vi "loading.vi"(10 "string2":string="勤眾興業", 11 "string1":string="CHEN") -> ()   [LabVIEW 2015]
uses:
  USER32.DLL
panel:
  in  "Color Box 2":u32(colorbox)=56466
  in  "CHEN 2":bool
  out "Cluster 11":T1
  in  "CHEN":bool
  in  "Color Box":u32(colorbox)=46079
  out "Cluster 10":T2
  out "Cluster 9":T3
  out "Cluster 8":T4
  out "Cluster 7":T3
  out "Cluster 6":T3
  out "Cluster 3":T3
  out "Cluster 4":T5
  out "Cluster 2":T6
  out "Cluster":T7
  out "Round Color Box 48":u32(colorbox)
  out "Round Color Box 47":u32(colorbox)
  out "Round Color Box 46":u32(colorbox)
  out "Round Color Box 45":u32(colorbox)
  out "Round Color Box 44":u32(colorbox)
  out "Round Color Box 43":u32(colorbox)
  out "Round Color Box 42":u32(colorbox)
  out "Round Color Box 41":u32(colorbox)
  out "Round Color Box 40":u32(colorbox)
  out "Round Color Box 39":u32(colorbox)
  out "Round Color Box 38":u32(colorbox)
  out "Round Color Box 37":u32(colorbox)
  out "Round Color Box 36":u32(colorbox)
  out "Round Color Box 35":u32(colorbox)
  out "Round Color Box 34":u32(colorbox)
  out "Round Color Box 33":u32(colorbox)
  out "Round Color Box 32":u32(colorbox)
  out "Round Color Box 31":u32(colorbox)
  out "Round Color Box 30":u32(colorbox)
  out "Round Color Box 29":u32(colorbox)
  out "Round Color Box 28":u32(colorbox)
  out "Round Color Box 27":u32(colorbox)
  out "Round Color Box 26":u32(colorbox)
  out "Round Color Box 25":u32(colorbox)
  out "Round Color Box 24":u32(colorbox)
  out "Round Color Box 23":u32(colorbox)
  out "Round Color Box 22":u32(colorbox)
  out "Round Color Box 21":u32(colorbox)
  out "Round Color Box 20":u32(colorbox)
  out "Round Color Box 19":u32(colorbox)
  out "Round Color Box 18":u32(colorbox)
  out "Round Color Box 17":u32(colorbox)
  in  "stop":bool
  out "Round Color Box 16":u32(colorbox)
  out "Round Color Box 15":u32(colorbox)
  out "Round Color Box 14":u32(colorbox)
  out "Round Color Box 13":u32(colorbox)
  out "Round Color Box 12":u32(colorbox)
  out "Round Color Box 11":u32(colorbox)
  out "Round Color Box 10":u32(colorbox)
  out "Round Color Box 9":u32(colorbox)
  out "Round Color Box 8":u32(colorbox)
  out "Round Color Box 7":u32(colorbox)
  out "Round Color Box 6":u32(colorbox)
  out "Round Color Box 5":u32(colorbox)
  out "Round Color Box 4":u32(colorbox)
  out "Round Color Box 3":u32(colorbox)
  out "Round Color Box 2":u32(colorbox)
  out "Round Color Box":u32(colorbox)
  # "Loading..."
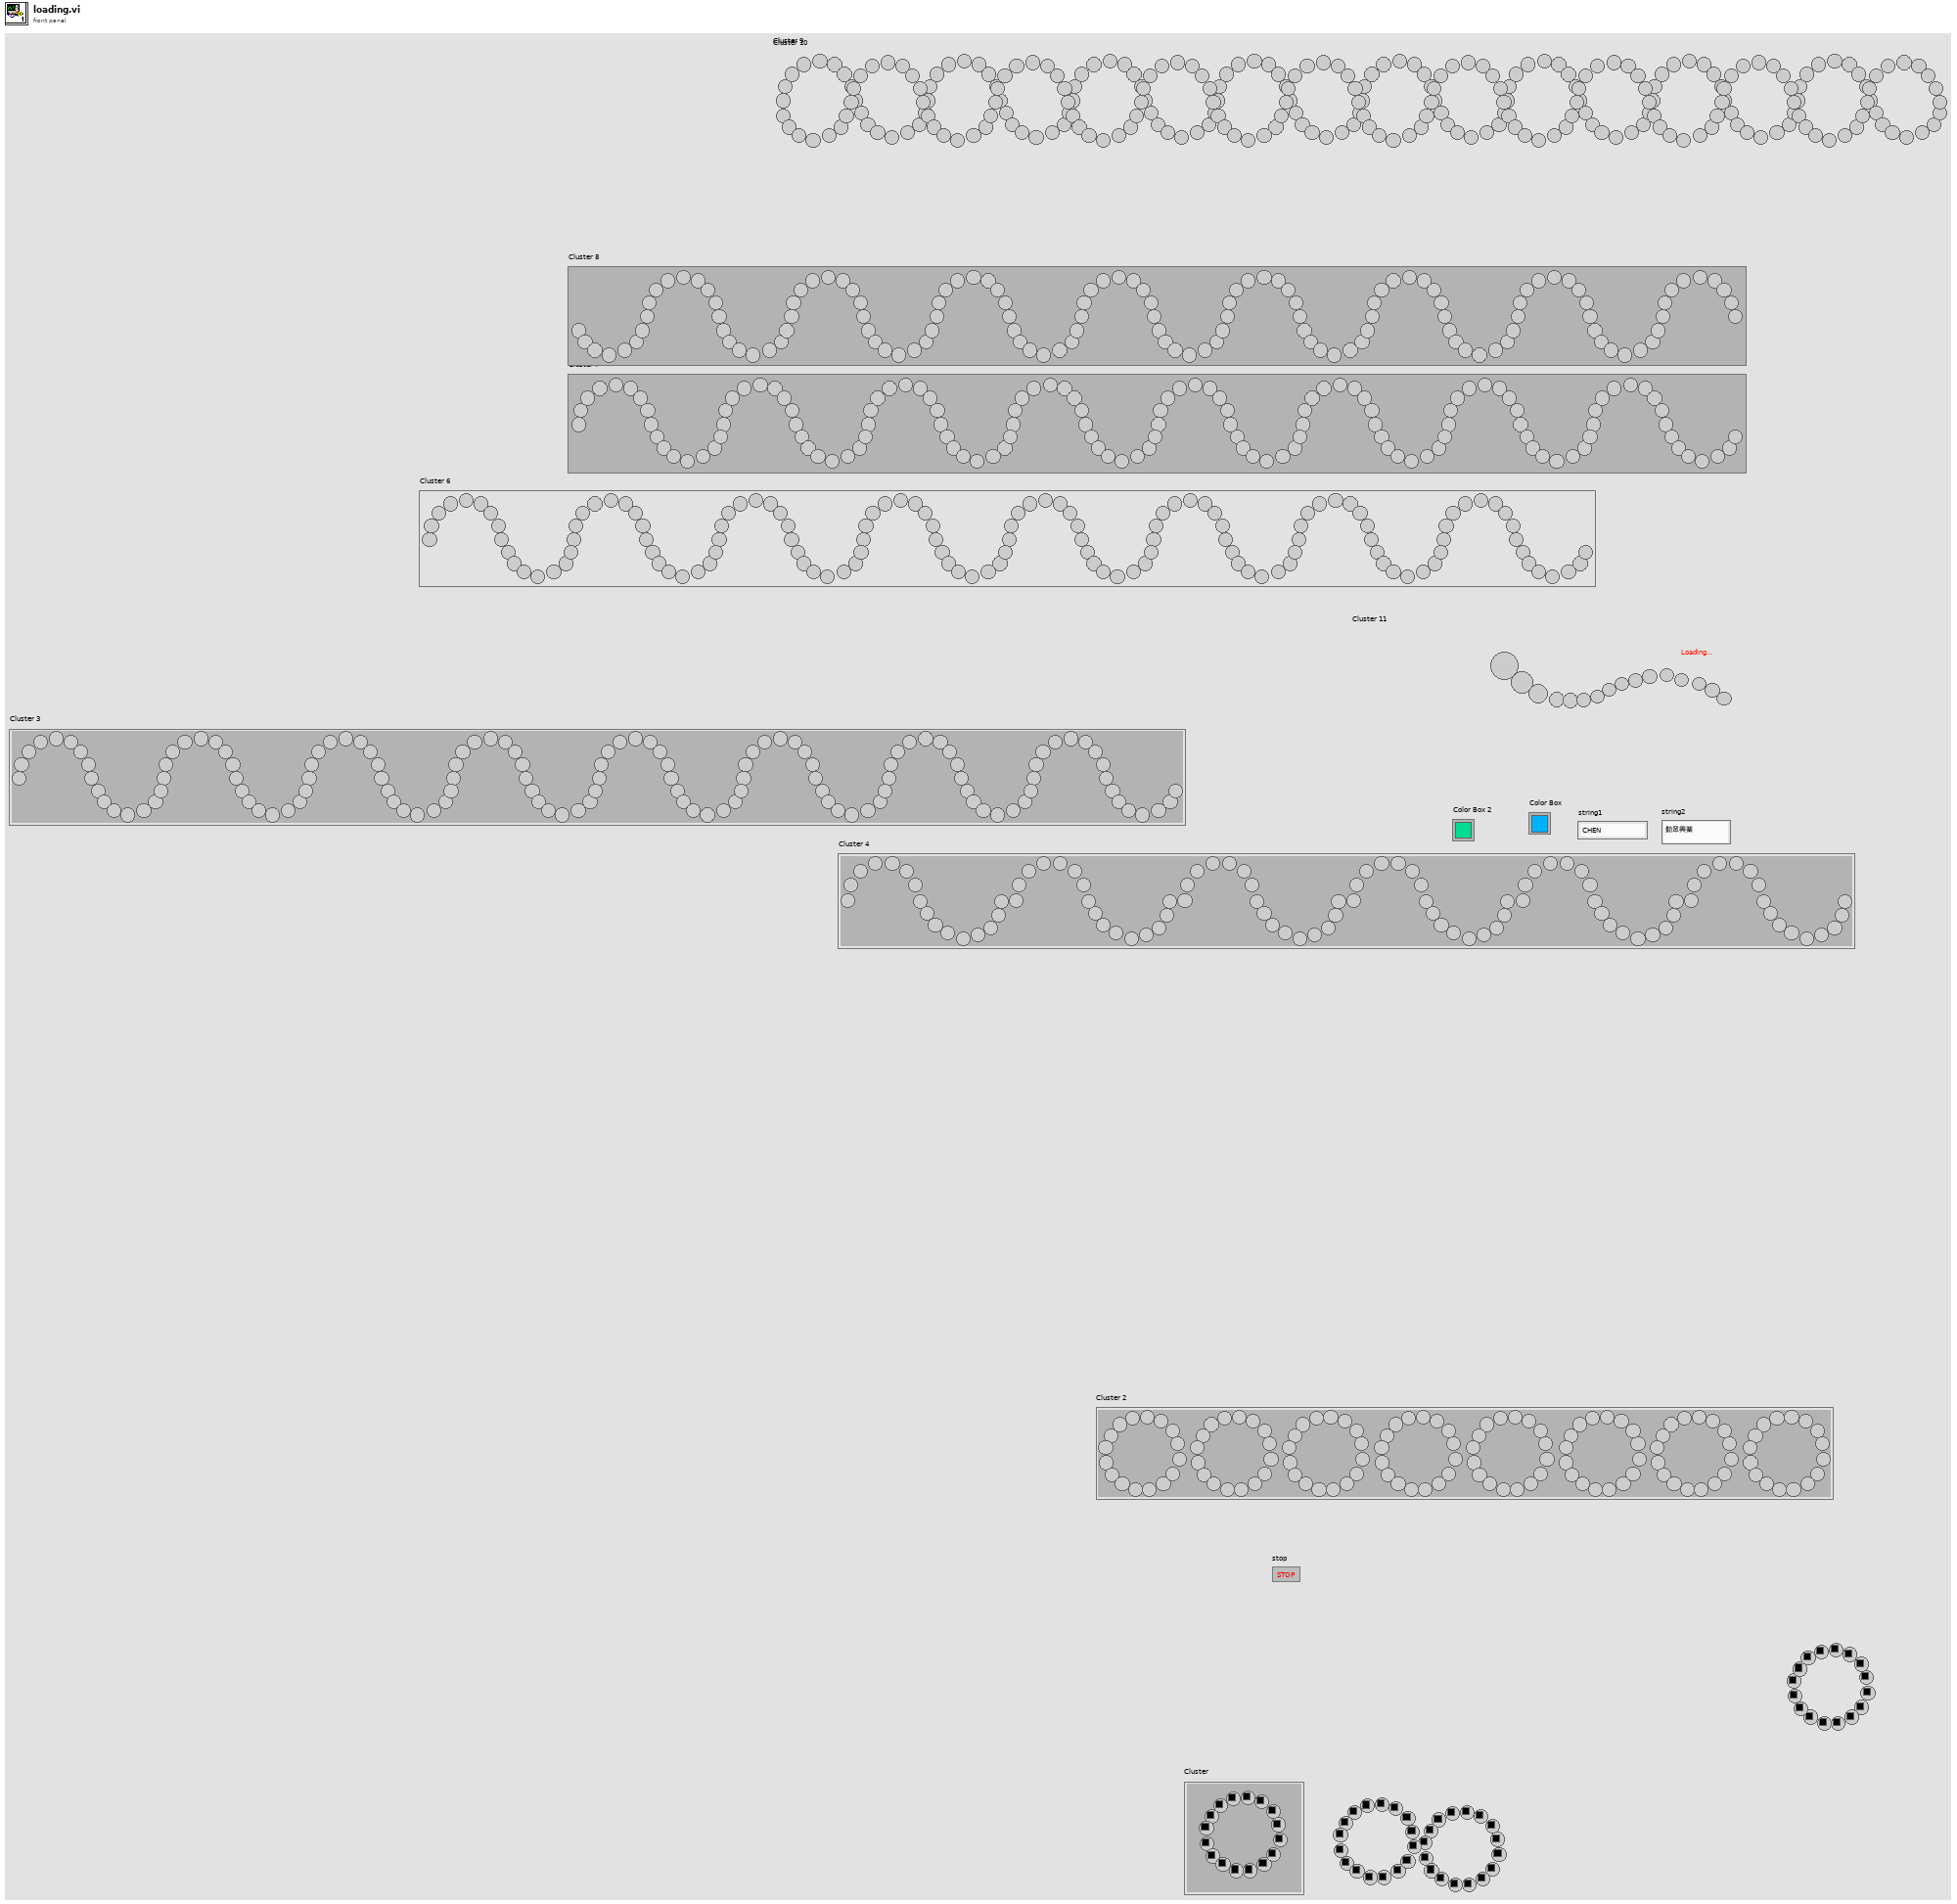
[diagram p1: front panel]
types:
  T1 = cluster{"Round Color Box 72":u32, "Round Color Box 73":u32, "Round Color Box 74":u32, "Round Color Box 75":u32, "Round Color Box 76":u32, "Round Color Box 77":u32, "Round Color Box 78":u32, "Round Color Box 79":u32, "Round Color Box 80":u32, "Round Color Box 65":u32, "Round Color Box 66":u32, "Round Color Box 67":u32, "Round Color Box 68":u32, "Round Color Box 69":u32, "Round Color Box 70":u32, "Round Color Box 71":u32}
  T2 = cluster{"Round Color Box 72":u32, "Round Color Box 73":u32, "Round Color Box 74":u32, "Round Color Box 75":u32, "Round Color Box 76":u32, "Round Color Box 77":u32, "Round Color Box 78":u32, "Round Color Box 79":u32, "Round Color Box 80":u32, "Round Color Box 65":u32, "Round Color Box 66":u32, "Round Color Box 67":u32, "Round Color Box 68":u32, "Round Color Box 69":u32, "Round Color Box 70":u32, "Round Color Box 71":u32, "Round Color Box 88":u32, "Round Color Box 89":u32, "Round Color Box 90":u32, "Round Color Box 91":u32, "Round Color Box 92":u32, "Round Color Box 93":u32, "Round Color Box 94":u32, "Round Color Box 95":u32, "Round Color Box 96":u32, "Round Color Box 81":u32, "Round Color Box 82":u32, "Round Color Box 83":u32, "Round Color Box 84":u32, "Round Color Box 85":u32, "Round Color Box 86":u32, "Round Color Box 87":u32, "Round Color Box 104":u32, "Round Color Box 105":u32, "Round Color Box 106":u32, "Round Color Box 107":u32, "Round Color Box 108":u32, "Round Color Box 109":u32, "Round Color Box 110":u32, "Round Color Box 111":u32, "Round Color Box 112":u32, "Round Color Box 97":u32, "Round Color Box 98":u32, "Round Color Box 99":u32, "Round Color Box 100":u32, "Round Color Box 101":u32, "Round Color Box 102":u32, "Round Color Box 103":u32, "Round Color Box 120":u32, "Round Color Box 121":u32, "Round Color Box 122":u32, "Round Color Box 123":u32, "Round Color Box 124":u32, "Round Color Box 125":u32, "Round Color Box 126":u32, "Round Color Box 127":u32, "Round Color Box 128":u32, "Round Color Box 113":u32, "Round Color Box 114":u32, "Round Color Box 115":u32, "Round Color Box 116":u32, "Round Color Box 117":u32, "Round Color Box 118":u32, "Round Color Box 119":u32, "Round Color Box 136":u32, "Round Color Box 137":u32, "Round Color Box 138":u32, "Round Color Box 139":u32, "Round Color Box 140":u32, "Round Color Box 141":u32, "Round Color Box 142":u32, "Round Color Box 143":u32, "Round Color Box 144":u32, "Round Color Box 129":u32, "Round Color Box 130":u32, "Round Color Box 131":u32, "Round Color Box 132":u32, "Round Color Box 133":u32, "Round Color Box 134":u32, "Round Color Box 135":u32, "Round Color Box 152":u32, "Round Color Box 153":u32, "Round Color Box 154":u32, "Round Color Box 155":u32, "Round Color Box 156":u32, "Round Color Box 157":u32, "Round Color Box 158":u32, "Round Color Box 159":u32, "Round Color Box 160":u32, "Round Color Box 145":u32, "Round Color Box 146":u32, "Round Color Box 147":u32, "Round Color Box 148":u32, "Round Color Box 149":u32, "Round Color Box 150":u32, "Round Color Box 151":u32, "Round Color Box 168":u32, "Round Color Box 169":u32, "Round Color Box 170":u32, "Round Color Box 171":u32, "Round Color Box 172":u32, "Round Color Box 173":u32, "Round Color Box 174":u32, "Round Color Box 175":u32, "Round Color Box 176":u32, "Round Color Box 161":u32, "Round Color Box 162":u32, "Round Color Box 163":u32, "Round Color Box 164":u32, "Round Color Box 165":u32, "Round Color Box 166":u32, "Round Color Box 167":u32, "Round Color Box 184":u32, "Round Color Box 185":u32, "Round Color Box 186":u32, "Round Color Box 187":u32, "Round Color Box 188":u32, "Round Color Box 189":u32, "Round Color Box 190":u32, "Round Color Box 191":u32, "Round Color Box 192":u32, "Round Color Box 177":u32, "Round Color Box 178":u32, "Round Color Box 179":u32, "Round Color Box 180":u32, "Round Color Box 181":u32, "Round Color Box 182":u32, "Round Color Box 183":u32}
  T3 = cluster{"Round Color Box 60":u32, "Round Color Box 59":u32, "Round Color Box 58":u32, "Round Color Box 57":u32, "Round Color Box 56":u32, "Round Color Box 55":u32, "Round Color Box 54":u32, "Round Color Box 53":u32, "Round Color Box 52":u32, "Round Color Box 51":u32, "Round Color Box 50":u32, "Round Color Box 49":u32, "Round Color Box 64":u32, "Round Color Box 63":u32, "Round Color Box 62":u32, "Round Color Box 61":u32, "Round Color Box 65":u32, "Round Color Box 66":u32, "Round Color Box 67":u32, "Round Color Box 68":u32, "Round Color Box 69":u32, "Round Color Box 70":u32, "Round Color Box 71":u32, "Round Color Box 72":u32, "Round Color Box 73":u32, "Round Color Box 74":u32, "Round Color Box 75":u32, "Round Color Box 76":u32, "Round Color Box 77":u32, "Round Color Box 78":u32, "Round Color Box 79":u32, "Round Color Box 80":u32, "Round Color Box 81":u32, "Round Color Box 82":u32, "Round Color Box 83":u32, "Round Color Box 84":u32, "Round Color Box 85":u32, "Round Color Box 86":u32, "Round Color Box 87":u32, "Round Color Box 88":u32, "Round Color Box 89":u32, "Round Color Box 90":u32, "Round Color Box 91":u32, "Round Color Box 92":u32, "Round Color Box 93":u32, "Round Color Box 94":u32, "Round Color Box 95":u32, "Round Color Box 96":u32, "Round Color Box 97":u32, "Round Color Box 98":u32, "Round Color Box 99":u32, "Round Color Box 100":u32, "Round Color Box 101":u32, "Round Color Box 102":u32, "Round Color Box 103":u32, "Round Color Box 104":u32, "Round Color Box 105":u32, "Round Color Box 106":u32, "Round Color Box 107":u32, "Round Color Box 108":u32, "Round Color Box 109":u32, "Round Color Box 110":u32, "Round Color Box 111":u32, "Round Color Box 112":u32, "Round Color Box 113":u32, "Round Color Box 114":u32, "Round Color Box 115":u32, "Round Color Box 116":u32, "Round Color Box 117":u32, "Round Color Box 118":u32, "Round Color Box 119":u32, "Round Color Box 120":u32, "Round Color Box 121":u32, "Round Color Box 122":u32, "Round Color Box 123":u32, "Round Color Box 124":u32, "Round Color Box 125":u32, "Round Color Box 126":u32, "Round Color Box 127":u32, "Round Color Box 128":u32, "Round Color Box 129":u32, "Round Color Box 130":u32, "Round Color Box 131":u32, "Round Color Box 132":u32, "Round Color Box 133":u32, "Round Color Box 134":u32, "Round Color Box 135":u32, "Round Color Box 136":u32, "Round Color Box 137":u32, "Round Color Box 138":u32, "Round Color Box 139":u32, "Round Color Box 140":u32, "Round Color Box 141":u32, "Round Color Box 142":u32, "Round Color Box 143":u32, "Round Color Box 144":u32, "Round Color Box 145":u32, "Round Color Box 146":u32, "Round Color Box 147":u32, "Round Color Box 148":u32, "Round Color Box 149":u32, "Round Color Box 150":u32, "Round Color Box 151":u32, "Round Color Box 152":u32, "Round Color Box 153":u32, "Round Color Box 154":u32, "Round Color Box 155":u32, "Round Color Box 156":u32, "Round Color Box 157":u32, "Round Color Box 158":u32, "Round Color Box 159":u32, "Round Color Box 160":u32, "Round Color Box 161":u32, "Round Color Box 162":u32, "Round Color Box 163":u32, "Round Color Box 164":u32, "Round Color Box 165":u32, "Round Color Box 166":u32, "Round Color Box 167":u32, "Round Color Box 168":u32, "Round Color Box 169":u32, "Round Color Box 170":u32, "Round Color Box 171":u32, "Round Color Box 172":u32, "Round Color Box 173":u32, "Round Color Box 174":u32, "Round Color Box 175":u32, "Round Color Box 176":u32}
  T4 = cluster{"Round Color Box 72":u32, "Round Color Box 73":u32, "Round Color Box 74":u32, "Round Color Box 75":u32, "Round Color Box 76":u32, "Round Color Box 77":u32, "Round Color Box 78":u32, "Round Color Box 79":u32, "Round Color Box 80":u32, "Round Color Box 65":u32, "Round Color Box 66":u32, "Round Color Box 67":u32, "Round Color Box 68":u32, "Round Color Box 69":u32, "Round Color Box 70":u32, "Round Color Box 71":u32, "Round Color Box 81":u32, "Round Color Box 82":u32, "Round Color Box 83":u32, "Round Color Box 84":u32, "Round Color Box 85":u32, "Round Color Box 86":u32, "Round Color Box 87":u32, "Round Color Box 88":u32, "Round Color Box 89":u32, "Round Color Box 90":u32, "Round Color Box 91":u32, "Round Color Box 92":u32, "Round Color Box 93":u32, "Round Color Box 94":u32, "Round Color Box 95":u32, "Round Color Box 96":u32, "Round Color Box 97":u32, "Round Color Box 98":u32, "Round Color Box 99":u32, "Round Color Box 100":u32, "Round Color Box 101":u32, "Round Color Box 102":u32, "Round Color Box 103":u32, "Round Color Box 104":u32, "Round Color Box 105":u32, "Round Color Box 106":u32, "Round Color Box 107":u32, "Round Color Box 108":u32, "Round Color Box 109":u32, "Round Color Box 110":u32, "Round Color Box 111":u32, "Round Color Box 112":u32, "Round Color Box 113":u32, "Round Color Box 114":u32, "Round Color Box 115":u32, "Round Color Box 116":u32, "Round Color Box 117":u32, "Round Color Box 118":u32, "Round Color Box 119":u32, "Round Color Box 120":u32, "Round Color Box 121":u32, "Round Color Box 122":u32, "Round Color Box 123":u32, "Round Color Box 124":u32, "Round Color Box 125":u32, "Round Color Box 126":u32, "Round Color Box 127":u32, "Round Color Box 128":u32, "Round Color Box 129":u32, "Round Color Box 130":u32, "Round Color Box 131":u32, "Round Color Box 132":u32, "Round Color Box 133":u32, "Round Color Box 134":u32, "Round Color Box 135":u32, "Round Color Box 136":u32, "Round Color Box 137":u32, "Round Color Box 138":u32, "Round Color Box 139":u32, "Round Color Box 140":u32, "Round Color Box 141":u32, "Round Color Box 142":u32, "Round Color Box 143":u32, "Round Color Box 144":u32, "Round Color Box 145":u32, "Round Color Box 146":u32, "Round Color Box 147":u32, "Round Color Box 148":u32, "Round Color Box 149":u32, "Round Color Box 150":u32, "Round Color Box 151":u32, "Round Color Box 152":u32, "Round Color Box 153":u32, "Round Color Box 154":u32, "Round Color Box 155":u32, "Round Color Box 156":u32, "Round Color Box 157":u32, "Round Color Box 158":u32, "Round Color Box 159":u32, "Round Color Box 160":u32, "Round Color Box 161":u32, "Round Color Box 162":u32, "Round Color Box 163":u32, "Round Color Box 164":u32, "Round Color Box 165":u32, "Round Color Box 166":u32, "Round Color Box 167":u32, "Round Color Box 168":u32, "Round Color Box 169":u32, "Round Color Box 170":u32, "Round Color Box 171":u32, "Round Color Box 172":u32, "Round Color Box 173":u32, "Round Color Box 174":u32, "Round Color Box 175":u32, "Round Color Box 176":u32, "Round Color Box 177":u32, "Round Color Box 178":u32, "Round Color Box 179":u32, "Round Color Box 180":u32, "Round Color Box 181":u32, "Round Color Box 182":u32, "Round Color Box 183":u32, "Round Color Box 184":u32, "Round Color Box 185":u32, "Round Color Box 186":u32, "Round Color Box 187":u32, "Round Color Box 188":u32, "Round Color Box 189":u32, "Round Color Box 190":u32, "Round Color Box 191":u32, "Round Color Box 192":u32}
  T5 = cluster{"Round Color Box 65":u32, "Round Color Box 66":u32, "Round Color Box 67":u32, "Round Color Box 68":u32, "Round Color Box 69":u32, "Round Color Box 70":u32, "Round Color Box 71":u32, "Round Color Box 72":u32, "Round Color Box 73":u32, "Round Color Box 74":u32, "Round Color Box 75":u32, "Round Color Box 76":u32, "Round Color Box 77":u32, "Round Color Box 78":u32, "Round Color Box 79":u32, "Round Color Box 80":u32, "Round Color Box 81":u32, "Round Color Box 82":u32, "Round Color Box 83":u32, "Round Color Box 84":u32, "Round Color Box 85":u32, "Round Color Box 86":u32, "Round Color Box 87":u32, "Round Color Box 88":u32, "Round Color Box 89":u32, "Round Color Box 90":u32, "Round Color Box 91":u32, "Round Color Box 92":u32, "Round Color Box 93":u32, "Round Color Box 94":u32, "Round Color Box 95":u32, "Round Color Box 96":u32, "Round Color Box 97":u32, "Round Color Box 98":u32, "Round Color Box 99":u32, "Round Color Box 100":u32, "Round Color Box 101":u32, "Round Color Box 102":u32, "Round Color Box 103":u32, "Round Color Box 104":u32, "Round Color Box 105":u32, "Round Color Box 106":u32, "Round Color Box 107":u32, "Round Color Box 108":u32, "Round Color Box 109":u32, "Round Color Box 110":u32, "Round Color Box 111":u32, "Round Color Box 112":u32, "Round Color Box 113":u32, "Round Color Box 114":u32, "Round Color Box 115":u32, "Round Color Box 116":u32, "Round Color Box 117":u32, "Round Color Box 118":u32, "Round Color Box 119":u32, "Round Color Box 120":u32, "Round Color Box 121":u32, "Round Color Box 122":u32, "Round Color Box 123":u32, "Round Color Box 124":u32, "Round Color Box 125":u32, "Round Color Box 126":u32, "Round Color Box 127":u32, "Round Color Box 128":u32, "Round Color Box 129":u32, "Round Color Box 130":u32, "Round Color Box 131":u32, "Round Color Box 132":u32, "Round Color Box 133":u32, "Round Color Box 134":u32, "Round Color Box 135":u32, "Round Color Box 136":u32, "Round Color Box 137":u32, "Round Color Box 138":u32, "Round Color Box 139":u32, "Round Color Box 140":u32, "Round Color Box 141":u32, "Round Color Box 142":u32, "Round Color Box 143":u32, "Round Color Box 144":u32, "Round Color Box 145":u32, "Round Color Box 146":u32, "Round Color Box 147":u32, "Round Color Box 148":u32, "Round Color Box 149":u32, "Round Color Box 150":u32, "Round Color Box 151":u32, "Round Color Box 152":u32, "Round Color Box 153":u32, "Round Color Box 154":u32, "Round Color Box 155":u32, "Round Color Box 156":u32, "Round Color Box 157":u32, "Round Color Box 158":u32, "Round Color Box 159":u32, "Round Color Box 160":u32}
  T6 = cluster{"Round Color Box 49":u32, "Round Color Box 50":u32, "Round Color Box 51":u32, "Round Color Box 52":u32, "Round Color Box 53":u32, "Round Color Box 54":u32, "Round Color Box 55":u32, "Round Color Box 56":u32, "Round Color Box 57":u32, "Round Color Box 58":u32, "Round Color Box 59":u32, "Round Color Box 60":u32, "Round Color Box 61":u32, "Round Color Box 62":u32, "Round Color Box 63":u32, "Round Color Box 64":u32, "Round Color Box 65":u32, "Round Color Box 66":u32, "Round Color Box 67":u32, "Round Color Box 68":u32, "Round Color Box 69":u32, "Round Color Box 70":u32, "Round Color Box 71":u32, "Round Color Box 72":u32, "Round Color Box 73":u32, "Round Color Box 74":u32, "Round Color Box 75":u32, "Round Color Box 76":u32, "Round Color Box 77":u32, "Round Color Box 78":u32, "Round Color Box 79":u32, "Round Color Box 80":u32, "Round Color Box 81":u32, "Round Color Box 82":u32, "Round Color Box 83":u32, "Round Color Box 84":u32, "Round Color Box 85":u32, "Round Color Box 86":u32, "Round Color Box 87":u32, "Round Color Box 88":u32, "Round Color Box 89":u32, "Round Color Box 90":u32, "Round Color Box 91":u32, "Round Color Box 92":u32, "Round Color Box 93":u32, "Round Color Box 94":u32, "Round Color Box 95":u32, "Round Color Box 96":u32, "Round Color Box 97":u32, "Round Color Box 98":u32, "Round Color Box 99":u32, "Round Color Box 100":u32, "Round Color Box 101":u32, "Round Color Box 102":u32, "Round Color Box 103":u32, "Round Color Box 104":u32, "Round Color Box 105":u32, "Round Color Box 106":u32, "Round Color Box 107":u32, "Round Color Box 108":u32, "Round Color Box 109":u32, "Round Color Box 110":u32, "Round Color Box 111":u32, "Round Color Box 112":u32, "Round Color Box 113":u32, "Round Color Box 114":u32, "Round Color Box 115":u32, "Round Color Box 116":u32, "Round Color Box 117":u32, "Round Color Box 118":u32, "Round Color Box 119":u32, "Round Color Box 120":u32, "Round Color Box 121":u32, "Round Color Box 122":u32, "Round Color Box 123":u32, "Round Color Box 124":u32, "Round Color Box 125":u32, "Round Color Box 126":u32, "Round Color Box 127":u32, "Round Color Box 128":u32, "Round Color Box 129":u32, "Round Color Box 130":u32, "Round Color Box 131":u32, "Round Color Box 132":u32, "Round Color Box 133":u32, "Round Color Box 134":u32, "Round Color Box 135":u32, "Round Color Box 136":u32, "Round Color Box 137":u32, "Round Color Box 138":u32, "Round Color Box 139":u32, "Round Color Box 140":u32, "Round Color Box 141":u32, "Round Color Box 142":u32, "Round Color Box 143":u32, "Round Color Box 144":u32, "Round Color Box 145":u32, "Round Color Box 146":u32, "Round Color Box 147":u32, "Round Color Box 148":u32, "Round Color Box 149":u32, "Round Color Box 150":u32, "Round Color Box 151":u32, "Round Color Box 152":u32, "Round Color Box 153":u32, "Round Color Box 154":u32, "Round Color Box 155":u32, "Round Color Box 156":u32, "Round Color Box 157":u32, "Round Color Box 158":u32, "Round Color Box 159":u32, "Round Color Box 160":u32, "Round Color Box 161":u32, "Round Color Box 162":u32, "Round Color Box 163":u32, "Round Color Box 164":u32, "Round Color Box 165":u32, "Round Color Box 166":u32, "Round Color Box 167":u32, "Round Color Box 168":u32, "Round Color Box 169":u32, "Round Color Box 170":u32, "Round Color Box 171":u32, "Round Color Box 172":u32, "Round Color Box 173":u32, "Round Color Box 174":u32, "Round Color Box 175":u32, "Round Color Box 176":u32}
  T7 = cluster{"Round Color Box 49":u32, "Round Color Box 50":u32, "Round Color Box 51":u32, "Round Color Box 52":u32, "Round Color Box 53":u32, "Round Color Box 54":u32, "Round Color Box 55":u32, "Round Color Box 56":u32, "Round Color Box 57":u32, "Round Color Box 58":u32, "Round Color Box 59":u32, "Round Color Box 60":u32, "Round Color Box 61":u32, "Round Color Box 62":u32, "Round Color Box 63":u32, "Round Color Box 64":u32}
  T8 = cluster{"Round Color Box":u32, "Round Color Box 2":u32, "Round Color Box 3":u32, "Round Color Box 4":u32, "Round Color Box 5":u32, "Round Color Box 6":u32, "Round Color Box 7":u32, "Round Color Box 8":u32, "Round Color Box 9":u32, "Round Color Box 10":u32, "Round Color Box 11":u32, "Round Color Box 12":u32, "Round Color Box 13":u32, "Round Color Box 14":u32, "Round Color Box 15":u32, "Round Color Box 16":u32}
  T9 = cluster{"[0]":u32, "[1]":u32, "[2]":u32, "[3]":u32, "[4]":u32, "[5]":u32, "[6]":u32, "[7]":u32, "[8]":u32, "[9]":u32, "[10]":u32, "[11]":u32, "[12]":u32, "[13]":u32, "[14]":u32, "[15]":u32}
  T10 = enum8{"Enabled", "Disabled", "Disabled and Grayed Out"}
  T11 = cluster{"[0]":u32, "[1]":u32, "[2]":u32, "[3]":u32, "[4]":u32, "[5]":u32, "[6]":u32, "[7]":u32, "[8]":u32, "[9]":u32, "[10]":u32, "[11]":u32, "[12]":u32, "[13]":u32, "[14]":u32, "[15]":u32, "[16]":u32, "[17]":u32, "[18]":u32, "[19]":u32, "[20]":u32, "[21]":u32, "[22]":u32, "[23]":u32, "[24]":u32, "[25]":u32, "[26]":u32, "[27]":u32, "[28]":u32, "[29]":u32, "[30]":u32, "[31]":u32, "[32]":u32, "[33]":u32, "[34]":u32, "[35]":u32, "[36]":u32, "[37]":u32, "[38]":u32, "[39]":u32, "[40]":u32, "[41]":u32, "[42]":u32, "[43]":u32, "[44]":u32, "[45]":u32, "[46]":u32, "[47]":u32, "[48]":u32, "[49]":u32, "[50]":u32, "[51]":u32, "[52]":u32, "[53]":u32, "[54]":u32, "[55]":u32, "[56]":u32, "[57]":u32, "[58]":u32, "[59]":u32, "[60]":u32, "[61]":u32, "[62]":u32, "[63]":u32, "[64]":u32, "[65]":u32, "[66]":u32, "[67]":u32, "[68]":u32, "[69]":u32, "[70]":u32, "[71]":u32, "[72]":u32, "[73]":u32, "[74]":u32, "[75]":u32, "[76]":u32, "[77]":u32, "[78]":u32, "[79]":u32, "[80]":u32, "[81]":u32, "[82]":u32, "[83]":u32, "[84]":u32, "[85]":u32, "[86]":u32, "[87]":u32, "[88]":u32, "[89]":u32, "[90]":u32, "[91]":u32, "[92]":u32, "[93]":u32, "[94]":u32, "[95]":u32, "[96]":u32, "[97]":u32, "[98]":u32, "[99]":u32, "[100]":u32, "[101]":u32, "[102]":u32, "[103]":u32, "[104]":u32, "[105]":u32, "[106]":u32, "[107]":u32, "[108]":u32, "[109]":u32, "[110]":u32, "[111]":u32, "[112]":u32, "[113]":u32, "[114]":u32, "[115]":u32, "[116]":u32, "[117]":u32, "[118]":u32, "[119]":u32, "[120]":u32, "[121]":u32, "[122]":u32, "[123]":u32, "[124]":u32, "[125]":u32, "[126]":u32, "[127]":u32}
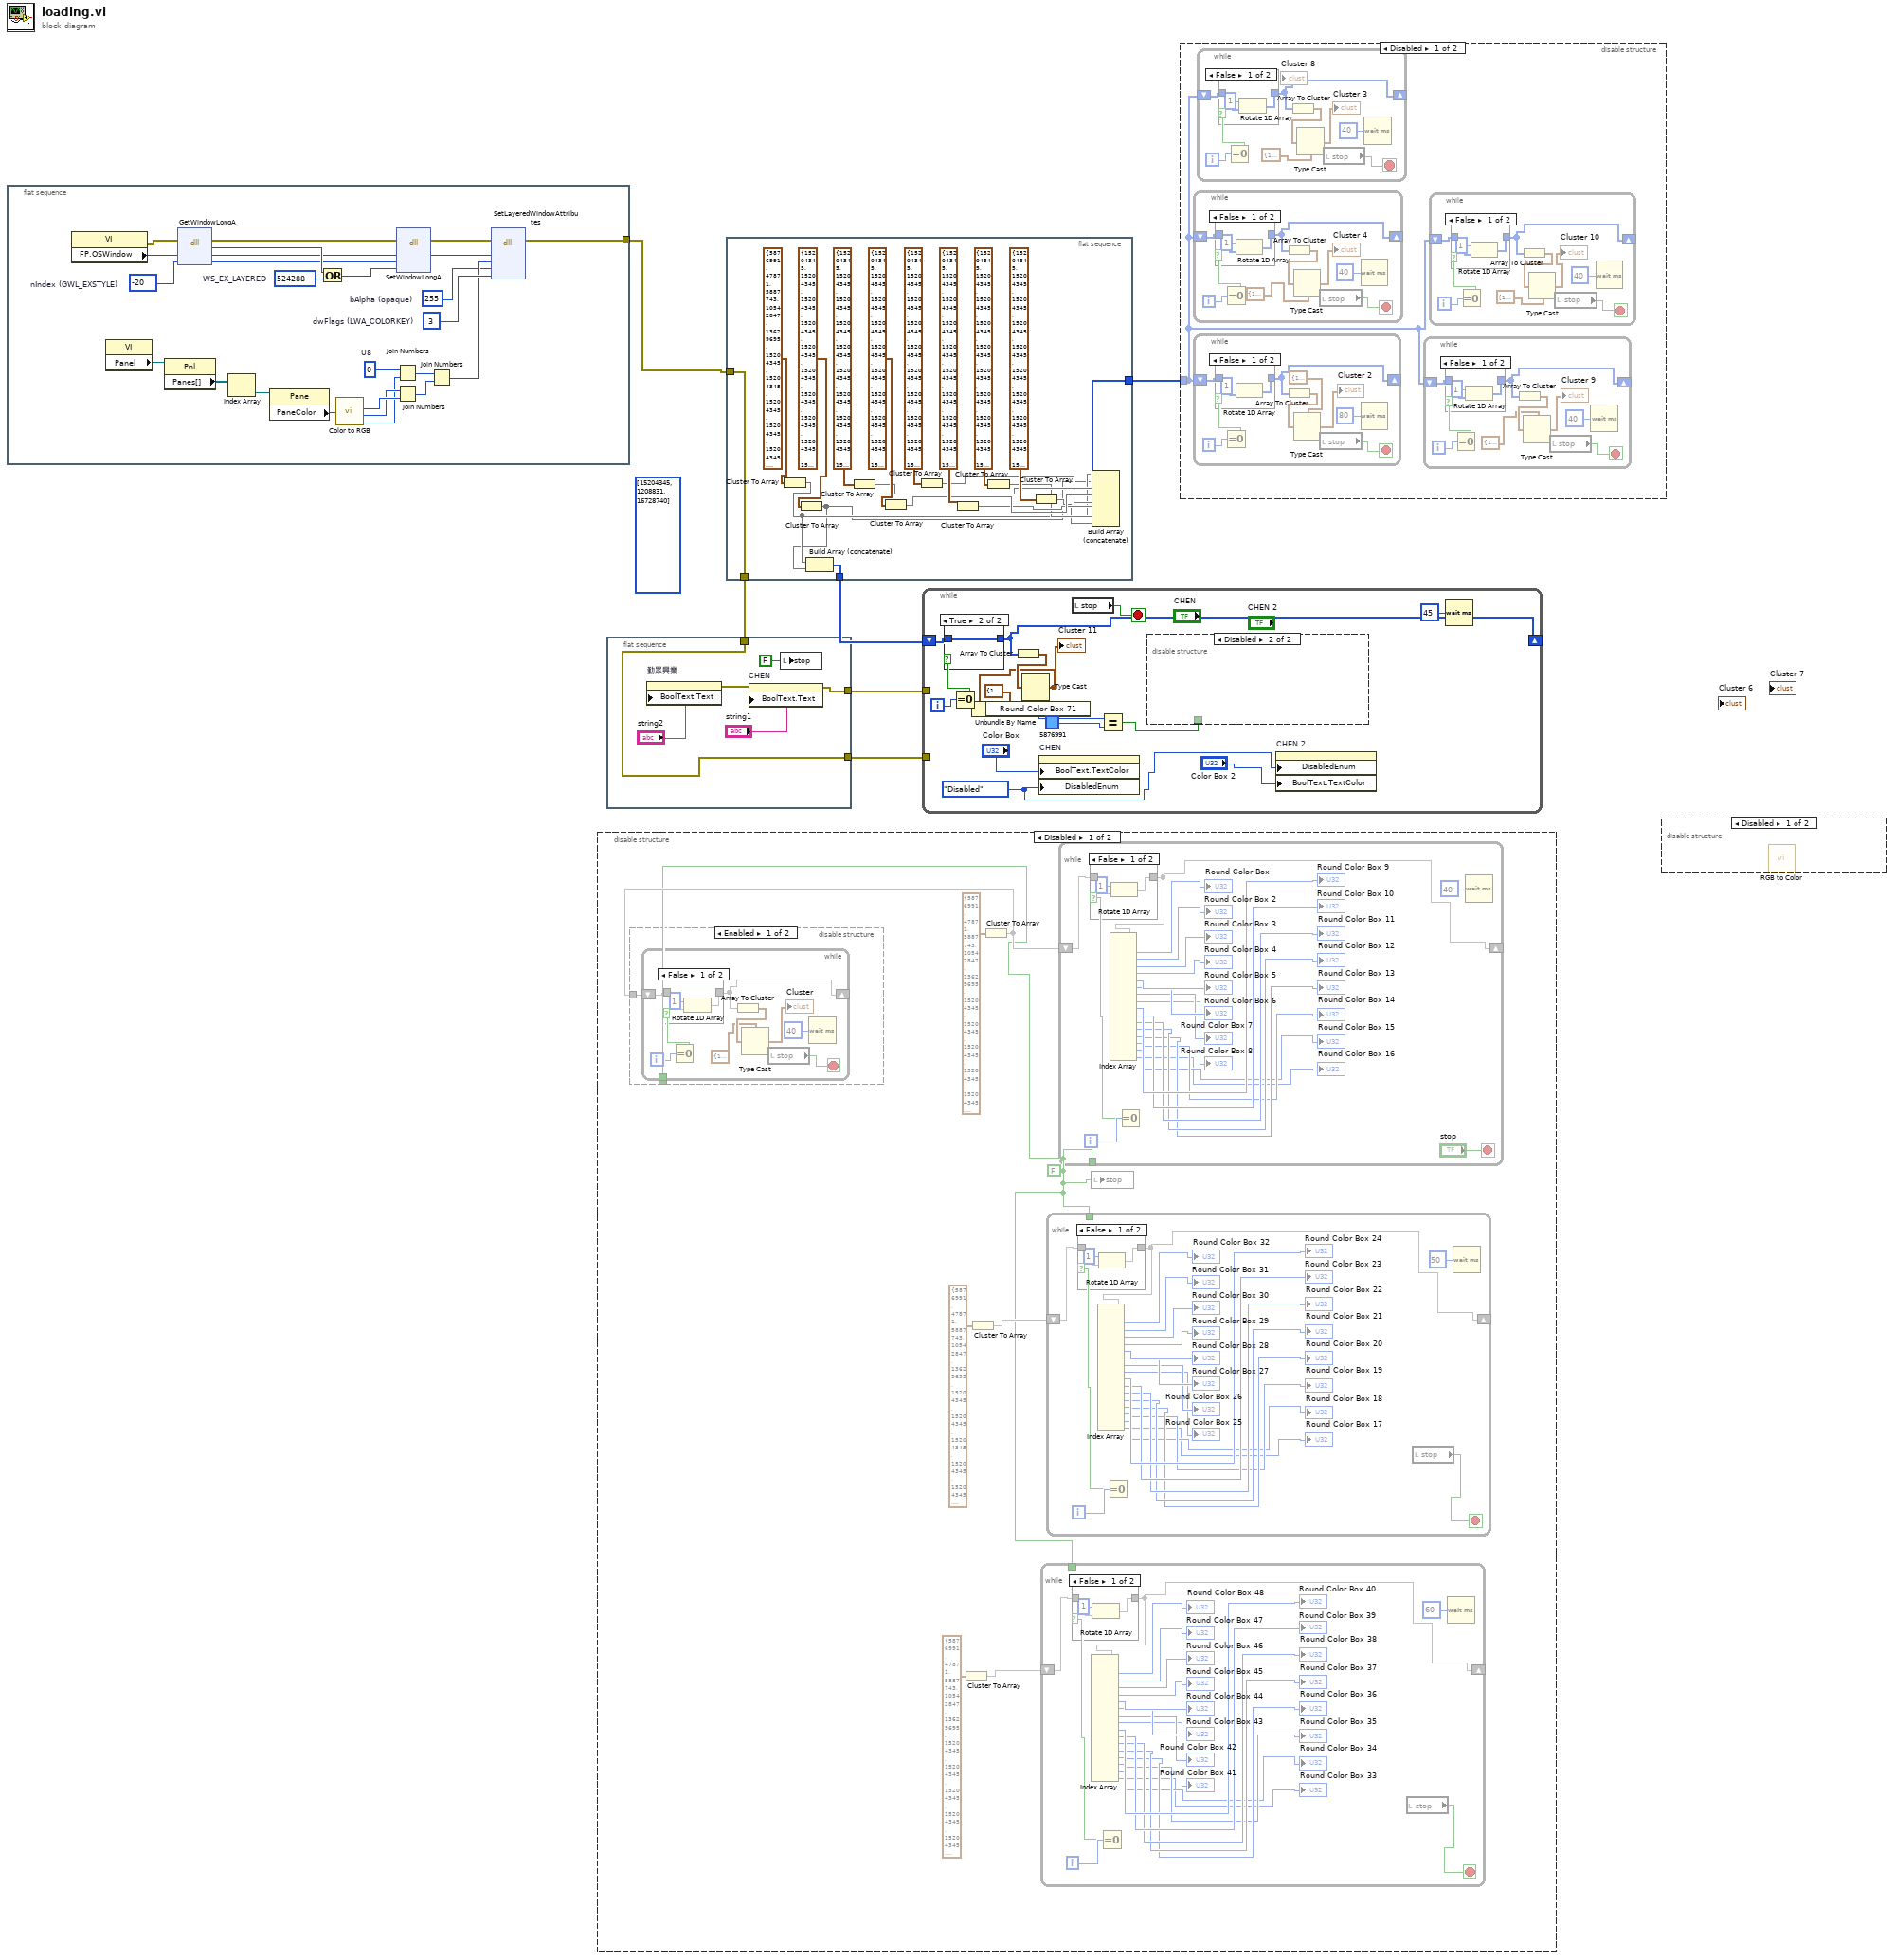
[diagram p0: block diagram]
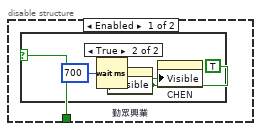
[diagram p14: hidden frame]
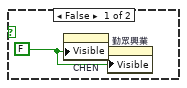
[diagram p15: hidden frame]
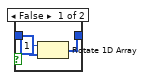
[diagram p16: hidden frame]
diagram:
  (unwired) u32[] [15204345, 1208831, 16728740]
  n1 = flat-sequence {
    tunnel: [w7] -> w3
    frame #0 {
      w20 = 524288  # WS_EX_LAYERED
      w17 = -20  # nIndex (GWL_EXSTYLE)
      w23 = 255  # bAlpha (opaque)
      w24 = u8 0  # U8
      w28 = 3  # dwFlags (LWA_COLORKEY)
      n2 = property class="VI"() -> (error out=w15:errorcluster, "FP.OSWindow"=w19:i32)  [unwired: 2 in, 1 out]
      n3 = property class="VI"() -> ("Panel"=w31:refnum<vi>)  [unwired: 2 in, 2 out]
      n4 = property class="Pnl"(reference=w31) -> ("Panes[]"=w30:refnum<vi>[])  [unwired: 1 in, 2 out]
      n5 = dll-call lib="USER32.DLL" fn="GetWindowLongA" label="getWindowLong"(error in=w15, "handle"=w19, "nIndex"=w17) -> (error out=w14:errorcluster, w21:i32, "handle"=w18:i32, "nIndex"=w16:i32)  [unwired: 2 in, 1 out]
      n6 = Index Array(array=w30) -> (element=w29:refnum<vi>)  [unwired: 1 in]
      n7 = property class="Pane"(reference=w29) -> ("PaneColor"=w11:u32)  [unwired: 1 in, 2 out]
      n8 = Or(x=w21, y=w20) -> (x .or. y?=w22:i32)
      n9 = call <vilib>:"Color to RGB.vi"("Color"=w11) -> ("R"=w10:u8, "G"=w9:u8, "B"=w8:u8)  [unwired: 1 out]
      n10 = Join Numbers(hi=w24, lo=w8) -> ((hi.lo)=w26:u16)
      n11 = Join Numbers(hi=w9, lo=w10) -> ((hi.lo)=w27:u16)
      n12 = dll-call lib="USER32.DLL" fn="SetWindowLongA" label="SetWindowLong"(error in=w14, "handle"=w18, "nIndex"=w16, "dwNewLong"=w22) -> (error out=w13:errorcluster, "handle"=w12:i32)  [unwired: 4 in, 2 out]
      n13 = Join Numbers(hi=w26, lo=w27) -> ((hi.lo)=w25:u32)
      n14 = dll-call lib="USER32.DLL" fn="SetLayeredWindowAttributes" label="SetLayerdWindowAttributs"(error in=w13, "handle"=w12, "crkey"=w25, "bAlpha"=w23, "dwFlags"=w28) -> (error out=w7:errorcluster)  [unwired: 6 in, 2 out]
    }
  }
  n15 = disable-structure shown="Disabled" {
    frame Disabled {
      w32 = FALSE ("stop")
      n16 = Cluster To Array(cluster=T8 {"Round Color Box"=5876991, "Round Color Box 2"=47871, "Round Color Box 3"=5887743, "Round Color Box 4"=10542847, "Round Color Box 5"=13629695, "Round Color Box 6"=15204345, "Round Color Box 7"=15204345, "Round Color Box 8"=15204345, "Round Color Box 9"=15204345, "Round Color Box 10"=15204345, "Round Color Box 11"=15204345, "Round Color Box 12"=15204345, "Round Color Box 13"=15204345, "Round Color Box 14"=15204345, "Round Color Box 15"=15204345, "Round Color Box 16"=15204345}) -> (array=w34:u32[])
      n17 = Cluster To Array(cluster=T8 {"Round Color Box"=5876991, "Round Color Box 2"=47871, "Round Color Box 3"=5887743, "Round Color Box 4"=10542847, "Round Color Box 5"=13629695, "Round Color Box 6"=15204345, "Round Color Box 7"=15204345, "Round Color Box 8"=15204345, "Round Color Box 9"=15204345, "Round Color Box 10"=15204345, "Round Color Box 11"=15204345, "Round Color Box 12"=15204345, "Round Color Box 13"=15204345, "Round Color Box 14"=15204345, "Round Color Box 15"=15204345, "Round Color Box 16"=15204345}) -> (array=w37:u32[])
      n18 = Cluster To Array(cluster=T8 {"Round Color Box"=5876991, "Round Color Box 2"=47871, "Round Color Box 3"=5887743, "Round Color Box 4"=10542847, "Round Color Box 5"=13629695, "Round Color Box 6"=15204345, "Round Color Box 7"=15204345, "Round Color Box 8"=15204345, "Round Color Box 9"=15204345, "Round Color Box 10"=15204345, "Round Color Box 11"=15204345, "Round Color Box 12"=15204345, "Round Color Box 13"=15204345, "Round Color Box 14"=15204345, "Round Color Box 15"=15204345, "Round Color Box 16"=15204345}) -> (array=w33:u32[])
      n19 = disable-structure shown="Enabled" {
        disable-tunnel: w33 -> [w40 _]
        disable-tunnel: w32 -> [w39 _]
        frame Enabled {
          n20 = while {
            shift-right: [w46] -> _
            shift-left: w40 -> [w49]
            tunnel: w39 -> [_]
            i -> [w48]
            stop <- w42 stop-if-true
            n21 = Equal To 0?(x=w48) -> (x = 0?=w47:bool)
            n22 = case shown="False" w47 {
              tunnel: [w51 w53] -> w46
              tunnel: w49 -> [w52 w53]
              frame False {
                n23 = Rotate 1D Array(1:w52, 2:1 ("n")) -> (0:w51:u32[])
              }
              frame True {
              }
            }
            n24 = Array To Cluster(array=w46) -> (cluster=w45:T9)
            n25 = Type Cast(type=T7 {"Round Color Box 49"=15204345, "Round Color Box 50"=15204345, "Round Color Box 51"=15204345, "Round Color Box 52"=15204345, "Round Color Box 53"=15204345, "Round Color Box 54"=15204345, "Round Color Box 55"=15204345, "Round Color Box 56"=15204345, "Round Color Box 57"=15204345, "Round Color Box 58"=15204345, "Round Color Box 59"=15204345, "Round Color Box 60"=13629695, "Round Color Box 61"=10542847, "Round Color Box 62"=5887743, "Round Color Box 63"=47871, "Round Color Box 64"=5876991} ("Cluster"), x=w45) -> (*(type *) &x=→"Cluster":T7)
            n26 = local read "stop"() -> (w42:bool)
            n27 = Wait (ms)(milliseconds to wait=u32 40) -> ()  [unwired: 1 out]
          }
        }
        frame Disabled {
        }
      }
      n28 = while {
        shift-right: [w55] -> _
        shift-left: w34 -> [w56]
        tunnel: w32 -> [_]
        i -> [w75]
        stop <- w54 stop-if-true
        n29 = Equal To 0?(x=w75) -> (x = 0?=w74:bool)
        n30 = case shown="False" w74 {
          tunnel: [w77 w79] -> w55
          tunnel: w56 -> [w78 w79]
          frame False {
            n31 = Rotate 1D Array(1:w78, 2:1 ("n")) -> (0:w77:u32[])
          }
          frame True {
          }
        }
        n32 = Index Array(array=w55) -> (element #1=→"Round Color Box 48":u32, element #2=→"Round Color Box 47":u32, element #3=→"Round Color Box 46":u32, element #4=→"Round Color Box 45":u32, element #5=→"Round Color Box 44":u32, element #6=→"Round Color Box 43":u32, element #7=→"Round Color Box 42":u32, element #8=→"Round Color Box 41":u32, element #9=→"Round Color Box 40":u32, element #10=→"Round Color Box 39":u32, element #11=→"Round Color Box 38":u32, element #12=→"Round Color Box 37":u32, element #13=→"Round Color Box 36":u32, element #14=→"Round Color Box 35":u32, element #15=→"Round Color Box 34":u32, element #16=→"Round Color Box 33":u32)  [unwired: 16 in]
        n33 = local read "stop"() -> (w54:bool)
        n34 = Wait (ms)(milliseconds to wait=u32 60) -> ()  [unwired: 1 out]
      }
      n35 = while {
        shift-right: [w81] -> _
        shift-left: w37 -> [w82]
        tunnel: w32 -> [_]
        i -> [w101]
        stop <- w80 stop-if-true
        n36 = Equal To 0?(x=w101) -> (x = 0?=w100:bool)
        n37 = case shown="False" w100 {
          tunnel: [w103 w105] -> w81
          tunnel: w82 -> [w104 w105]
          frame False {
            n38 = Rotate 1D Array(1:w104, 2:1 ("n")) -> (0:w103:u32[])
          }
          frame True {
          }
        }
        n39 = Index Array(array=w81) -> (element #1=→"Round Color Box 32":u32, element #2=→"Round Color Box 31":u32, element #3=→"Round Color Box 30":u32, element #4=→"Round Color Box 29":u32, element #5=→"Round Color Box 28":u32, element #6=→"Round Color Box 27":u32, element #7=→"Round Color Box 26":u32, element #8=→"Round Color Box 25":u32, element #9=→"Round Color Box 24":u32, element #10=→"Round Color Box 23":u32, element #11=→"Round Color Box 22":u32, element #12=→"Round Color Box 21":u32, element #13=→"Round Color Box 20":u32, element #14=→"Round Color Box 19":u32, element #15=→"Round Color Box 18":u32, element #16=→"Round Color Box 17":u32)  [unwired: 16 in]
        n40 = local read "stop"() -> (w80:bool)
        n41 = Wait (ms)(milliseconds to wait=u32 50) -> ()  [unwired: 1 out]
      }
      n42 = while {
        shift-right: [w106] -> _
        shift-left: w33 -> [w107]
        tunnel: w32 -> [_]
        i -> [w127]
        stop <- "stop" stop-if-true
        n43 = Equal To 0?(x=w127) -> (x = 0?=w126:bool)
        n44 = case shown="False" w126 {
          tunnel: [w129 w131] -> w106
          tunnel: w107 -> [w130 w131]
          frame False {
            n45 = Rotate 1D Array(1:w130, 2:1 ("n")) -> (0:w129:u32[])
          }
          frame True {
          }
        }
        n46 = Index Array(array=w106) -> (element #1=→"Round Color Box":u32, element #2=→"Round Color Box 2":u32, element #3=→"Round Color Box 3":u32, element #4=→"Round Color Box 4":u32, element #5=→"Round Color Box 5":u32, element #6=→"Round Color Box 6":u32, element #7=→"Round Color Box 7":u32, element #8=→"Round Color Box 8":u32, element #9=→"Round Color Box 9":u32, element #10=→"Round Color Box 10":u32, element #11=→"Round Color Box 11":u32, element #12=→"Round Color Box 12":u32, element #13=→"Round Color Box 13":u32, element #14=→"Round Color Box 14":u32, element #15=→"Round Color Box 15":u32, element #16=→"Round Color Box 16":u32)  [unwired: 16 in]
        n47 = Wait (ms)(milliseconds to wait=u32 40) -> ()  [unwired: 1 out]
      }
      n48 = local write "stop"(w32) -> ()
    }
    frame Enabled {
    }
  }
  n49 = flat-sequence {
    tunnel: [w136] -> w4
    tunnel: w2 -> [w132]
    tunnel: [w132] -> w1
    frame #0 {
      n50 = property on="勤眾興業" class="Bool (strict)"("BoolText.Text"="string2") -> (error out=w137:errorcluster)  [unwired: 2 in, 1 out]
      n51 = property on="CHEN" class="Bool (strict)"(error in=w137, "BoolText.Text"="string1") -> (error out=w136:errorcluster)  [unwired: 1 in, 1 out]
      n52 = local write "stop"(FALSE ("stop")) -> ()
    }
  }
  n53 = flat-sequence {
    tunnel: [w142] -> w6
    tunnel: [w139] -> w5
    tunnel: w3 -> [w138]
    tunnel: [w138] -> w2
    frame #0 {
      n54 = Cluster To Array(cluster=T8 {"Round Color Box"=5876991, "Round Color Box 2"=47871, "Round Color Box 3"=5887743, "Round Color Box 4"=10542847, "Round Color Box 5"=13629695, "Round Color Box 6"=15204345, "Round Color Box 7"=15204345, "Round Color Box 8"=15204345, "Round Color Box 9"=15204345, "Round Color Box 10"=15204345, "Round Color Box 11"=15204345, "Round Color Box 12"=15204345, "Round Color Box 13"=15204345, "Round Color Box 14"=15204345, "Round Color Box 15"=15204345, "Round Color Box 16"=15204345}) -> (array=w141:u32[])
      n55 = Cluster To Array(cluster=T8 {"Round Color Box"=15204345, "Round Color Box 2"=15204345, "Round Color Box 3"=15204345, "Round Color Box 4"=15204345, "Round Color Box 5"=15204345, "Round Color Box 6"=15204345, "Round Color Box 7"=15204345, "Round Color Box 8"=15204345, "Round Color Box 9"=15204345, "Round Color Box 10"=15204345, "Round Color Box 11"=15204345, "Round Color Box 12"=15204345, "Round Color Box 13"=15204345, "Round Color Box 14"=15204345, "Round Color Box 15"=15204345, "Round Color Box 16"=15204345}) -> (array=w140:u32[])
      n56 = Build Array (concatenate)(w141, w140) -> (w139:u32[])
      n57 = Cluster To Array(cluster=T8 {"Round Color Box"=15204345, "Round Color Box 2"=15204345, "Round Color Box 3"=15204345, "Round Color Box 4"=15204345, "Round Color Box 5"=15204345, "Round Color Box 6"=15204345, "Round Color Box 7"=15204345, "Round Color Box 8"=15204345, "Round Color Box 9"=15204345, "Round Color Box 10"=15204345, "Round Color Box 11"=15204345, "Round Color Box 12"=15204345, "Round Color Box 13"=15204345, "Round Color Box 14"=15204345, "Round Color Box 15"=15204345, "Round Color Box 16"=15204345}) -> (array=w148:u32[])
      n58 = Cluster To Array(cluster=T8 {"Round Color Box"=15204345, "Round Color Box 2"=15204345, "Round Color Box 3"=15204345, "Round Color Box 4"=15204345, "Round Color Box 5"=15204345, "Round Color Box 6"=15204345, "Round Color Box 7"=15204345, "Round Color Box 8"=15204345, "Round Color Box 9"=15204345, "Round Color Box 10"=15204345, "Round Color Box 11"=15204345, "Round Color Box 12"=15204345, "Round Color Box 13"=15204345, "Round Color Box 14"=15204345, "Round Color Box 15"=15204345, "Round Color Box 16"=15204345}) -> (array=w147:u32[])
      n59 = Cluster To Array(cluster=T8 {"Round Color Box"=15204345, "Round Color Box 2"=15204345, "Round Color Box 3"=15204345, "Round Color Box 4"=15204345, "Round Color Box 5"=15204345, "Round Color Box 6"=15204345, "Round Color Box 7"=15204345, "Round Color Box 8"=15204345, "Round Color Box 9"=15204345, "Round Color Box 10"=15204345, "Round Color Box 11"=15204345, "Round Color Box 12"=15204345, "Round Color Box 13"=15204345, "Round Color Box 14"=15204345, "Round Color Box 15"=15204345, "Round Color Box 16"=15204345}) -> (array=w146:u32[])
      n60 = Cluster To Array(cluster=T8 {"Round Color Box"=15204345, "Round Color Box 2"=15204345, "Round Color Box 3"=15204345, "Round Color Box 4"=15204345, "Round Color Box 5"=15204345, "Round Color Box 6"=15204345, "Round Color Box 7"=15204345, "Round Color Box 8"=15204345, "Round Color Box 9"=15204345, "Round Color Box 10"=15204345, "Round Color Box 11"=15204345, "Round Color Box 12"=15204345, "Round Color Box 13"=15204345, "Round Color Box 14"=15204345, "Round Color Box 15"=15204345, "Round Color Box 16"=15204345}) -> (array=w145:u32[])
      n61 = Cluster To Array(cluster=T8 {"Round Color Box"=15204345, "Round Color Box 2"=15204345, "Round Color Box 3"=15204345, "Round Color Box 4"=15204345, "Round Color Box 5"=15204345, "Round Color Box 6"=15204345, "Round Color Box 7"=15204345, "Round Color Box 8"=15204345, "Round Color Box 9"=15204345, "Round Color Box 10"=15204345, "Round Color Box 11"=15204345, "Round Color Box 12"=15204345, "Round Color Box 13"=15204345, "Round Color Box 14"=15204345, "Round Color Box 15"=15204345, "Round Color Box 16"=15204345}) -> (array=w144:u32[])
      n62 = Cluster To Array(cluster=T8 {"Round Color Box"=15204345, "Round Color Box 2"=15204345, "Round Color Box 3"=15204345, "Round Color Box 4"=15204345, "Round Color Box 5"=15204345, "Round Color Box 6"=15204345, "Round Color Box 7"=15204345, "Round Color Box 8"=15204345, "Round Color Box 9"=15204345, "Round Color Box 10"=15204345, "Round Color Box 11"=15204345, "Round Color Box 12"=15204345, "Round Color Box 13"=15204345, "Round Color Box 14"=15204345, "Round Color Box 15"=15204345, "Round Color Box 16"=15204345}) -> (array=w143:u32[])
      n63 = Build Array (concatenate)(w141, w140, w148, w147, w146, w145, w144, w143) -> (w142:u32[])
    }
  }
  n64 = while {
    shift-right: [w168] -> _
    shift-left: w5 -> [w171]
    tunnel: w4 -> [_]
    tunnel: w1 -> [_]
    i -> [w170]
    stop <- w166 stop-if-true
    w157 = T10."Disabled" ("Disabled")
    n65 = Equal To 0?(x=w170) -> (x = 0?=w169:bool)
    n66 = case shown="True" w169 {
      tunnel: [w177 w179] -> w168
      tunnel: w171 -> [w178 w179]
      frame False {
        n67 = Rotate 1D Array(1:w178, 2:1 ("n")) -> (0:w177:u32[])
      }
      frame True {
      }
    }
    n68 = Array To Cluster(array=w168) -> (cluster=w167:T11)
    n69 = Type Cast(type=T1 {"Round Color Box 72"=10542847, "Round Color Box 73"=5887743, "Round Color Box 74"=47871, "Round Color Box 75"=5876991, "Round Color Box 76"=15204345, "Round Color Box 77"=15204345, "Round Color Box 78"=15204345, "Round Color Box 79"=15204345, "Round Color Box 80"=15204345, "Round Color Box 65"=15204345, "Round Color Box 66"=15204345, "Round Color Box 67"=15204345, "Round Color Box 68"=15204345, "Round Color Box 69"=15204345, "Round Color Box 70"=15204345, "Round Color Box 71"=13629695} ("Cluster 11"), x=w167) -> (*(type *) &x=w162:T1)
    "Cluster 11" <- w162
    n70 = Unbundle By Name(w162) -> ("Round Color Box 71"=w161:u32)
    n71 = property on="CHEN" class="Bool (strict)"("BoolText.TextColor"="Color Box", "DisabledEnum"=w157) -> ()  [unwired: 2 in, 2 out]
    n72 = local read "stop"() -> (w166:bool)
    n73 = Equal?(x=w161, y=u32 5876991 ("Round Color Box")) -> (x = y?=w159:bool)
    n74 = disable-structure shown="Disabled" {
      disable-tunnel: w159 -> [w172 _]
      frame Enabled {
        n75 = case shown="True" w172 {
          frame False {
            w173 = FALSE ("Visible")
            n76 = property on="CHEN" class="Bool (strict)"("Visible"=w173) -> ()  [unwired: 2 in, 2 out]
            n77 = property on="勤眾興業" class="Bool (strict)"("Visible"=w173) -> ()  [unwired: 2 in, 2 out]
          }
          frame True {
            w174 = TRUE ("Visible")
            n78 = Wait (ms)(milliseconds to wait=u32 700) -> ()  [unwired: 1 out]
            n79 = property on="勤眾興業" class="Bool (strict)"("Visible"=w174) -> ()  [unwired: 2 in, 2 out]
            n80 = property on="CHEN" class="Bool (strict)"("Visible"=w174) -> ()  [unwired: 2 in, 2 out]
          }
        }
      }
      frame Disabled {
      }
    }
    n81 = property on="CHEN 2" class="Bool (strict)"("DisabledEnum"=w157, "BoolText.TextColor"="Color Box 2") -> ()  [unwired: 2 in, 2 out]
    n82 = Wait (ms)(milliseconds to wait=u32 45) -> ()  [unwired: 1 out]
  }
  n83 = disable-structure shown="Disabled" {
    disable-tunnel: w6 -> [w180 _]
    frame Disabled {
      n84 = while {
        shift-right: [w225] -> _
        shift-left: w180 -> [w228]
        i -> [w227]
        stop <- w223 stop-if-true
        n85 = Equal To 0?(x=w227) -> (x = 0?=w226:bool)
        n86 = case shown="False" w226 {
          tunnel: [w230 w232] -> w225
          tunnel: w228 -> [w231 w232]
          frame False {
            n87 = Rotate 1D Array(1:w231, 2:1 ("n")) -> (0:w230:u32[])
          }
          frame True {
          }
        }
        n88 = Array To Cluster(array=w225) -> (cluster=w224:T11)
        n89 = Type Cast(type=T5 {"Round Color Box 65"=15204345, "Round Color Box 66"=15204345, "Round Color Box 67"=15204345, "Round Color Box 68"=15204345, "Round Color Box 69"=15204345, "Round Color Box 70"=15204345, "Round Color Box 71"=15204345, "Round Color Box 72"=15204345, "Round Color Box 73"=15204345, "Round Color Box 74"=15204345, "Round Color Box 75"=15204345, "Round Color Box 76"=15204345, "Round Color Box 77"=15204345, "Round Color Box 78"=15204345, "Round Color Box 79"=15204345, "Round Color Box 80"=15204345, "Round Color Box 81"=15204345, "Round Color Box 82"=15204345, "Round Color Box 83"=15204345, "Round Color Box 84"=15204345, "Round Color Box 85"=15204345, "Round Color Box 86"=15204345, "Round Color Box 87"=15204345, "Round Color Box 88"=15204345, "Round Color Box 89"=15204345, "Round Color Box 90"=15204345, "Round Color Box 91"=15204345, "Round Color Box 92"=15204345, "Round Color Box 93"=15204345, "Round Color Box 94"=15204345, "Round Color Box 95"=15204345, "Round Color Box 96"=15204345, "Round Color Box 97"=15204345, "Round Color Box 98"=15204345, "Round Color Box 99"=15204345, "Round Color Box 100"=15204345, "Round Color Box 101"=15204345, "Round Color Box 102"=15204345, "Round Color Box 103"=15204345, "Round Color Box 104"=15204345, "Round Color Box 105"=15204345, "Round Color Box 106"=15204345, "Round Color Box 107"=15204345, "Round Color Box 108"=15204345, "Round Color Box 109"=15204345, "Round Color Box 110"=15204345, "Round Color Box 111"=15204345, "Round Color Box 112"=15204345, "Round Color Box 113"=15204345, "Round Color Box 114"=15204345, "Round Color Box 115"=15204345, "Round Color Box 116"=15204345, "Round Color Box 117"=15204345, "Round Color Box 118"=15204345, "Round Color Box 119"=15204345, "Round Color Box 120"=15204345, "Round Color Box 121"=15204345, "Round Color Box 122"=15204345, "Round Color Box 123"=15204345, "Round Color Box 124"=15204345, "Round Color Box 125"=15204345, "Round Color Box 126"=15204345, "Round Color Box 127"=15204345, "Round Color Box 128"=15204345, "Round Color Box 129"=15204345, "Round Color Box 130"=15204345, "Round Color Box 131"=15204345, "Round Color Box 132"=15204345, "Round Color Box 133"=15204345, "Round Color Box 134"=15204345, "Round Color Box 135"=15204345, "Round Color Box 136"=15204345, "Round Color Box 137"=15204345, "Round Color Box 138"=15204345, "Round Color Box 139"=15204345, "Round Color Box 140"=15204345, "Round Color Box 141"=15204345, "Round Color Box 142"=15204345, "Round Color Box 143"=15204345, "Round Color Box 144"=15204345, "Round Color Box 145"=15204345, "Round Color Box 146"=15204345, "Round Color Box 147"=15204345, "Round Color Box 148"=15204345, "Round Color Box 149"=15204345, "Round Color Box 150"=15204345, "Round Color Box 151"=15204345, "Round Color Box 152"=15204345, "Round Color Box 153"=15204345, "Round Color Box 154"=15204345, "Round Color Box 155"=15204345, "Round Color Box 156"=15204345, "Round Color Box 157"=15204345, "Round Color Box 158"=15204345, "Round Color Box 159"=15204345, "Round Color Box 160"=15204345} ("Cluster 4"), x=w224) -> (*(type *) &x=→"Cluster 4":T5)
        n90 = local read "stop"() -> (w223:bool)
        n91 = Wait (ms)(milliseconds to wait=u32 40) -> ()  [unwired: 1 out]
      }
      n92 = while {
        shift-right: [w238] -> _
        shift-left: w180 -> [w241]
        i -> [w240]
        stop <- w236 stop-if-true
        n93 = Equal To 0?(x=w240) -> (x = 0?=w239:bool)
        n94 = case shown="False" w239 {
          tunnel: [w243 w245] -> w238
          tunnel: w241 -> [w244 w245]
          frame False {
            n95 = Rotate 1D Array(1:w244, 2:1 ("n")) -> (0:w243:u32[])
          }
          frame True {
          }
        }
        n96 = Array To Cluster(array=w238) -> (cluster=w237:T11)
        n97 = Type Cast(type=T6 {"Round Color Box 49"=15204345, "Round Color Box 50"=15204345, "Round Color Box 51"=15204345, "Round Color Box 52"=15204345, "Round Color Box 53"=15204345, "Round Color Box 54"=15204345, "Round Color Box 55"=15204345, "Round Color Box 56"=15204345, "Round Color Box 57"=15204345, "Round Color Box 58"=15204345, "Round Color Box 59"=15204345, "Round Color Box 60"=15204345, "Round Color Box 61"=15204345, "Round Color Box 62"=15204345, "Round Color Box 63"=15204345, "Round Color Box 64"=15204345, "Round Color Box 65"=15204345, "Round Color Box 66"=15204345, "Round Color Box 67"=15204345, "Round Color Box 68"=15204345, "Round Color Box 69"=15204345, "Round Color Box 70"=15204345, "Round Color Box 71"=15204345, "Round Color Box 72"=15204345, "Round Color Box 73"=15204345, "Round Color Box 74"=15204345, "Round Color Box 75"=15204345, "Round Color Box 76"=15204345, "Round Color Box 77"=15204345, "Round Color Box 78"=15204345, "Round Color Box 79"=15204345, "Round Color Box 80"=15204345, "Round Color Box 81"=15204345, "Round Color Box 82"=15204345, "Round Color Box 83"=15204345, "Round Color Box 84"=15204345, "Round Color Box 85"=15204345, "Round Color Box 86"=15204345, "Round Color Box 87"=15204345, "Round Color Box 88"=15204345, "Round Color Box 89"=15204345, "Round Color Box 90"=15204345, "Round Color Box 91"=15204345, "Round Color Box 92"=15204345, "Round Color Box 93"=15204345, "Round Color Box 94"=15204345, "Round Color Box 95"=15204345, "Round Color Box 96"=15204345, "Round Color Box 97"=15204345, "Round Color Box 98"=15204345, "Round Color Box 99"=15204345, "Round Color Box 100"=15204345, "Round Color Box 101"=15204345, "Round Color Box 102"=15204345, "Round Color Box 103"=15204345, "Round Color Box 104"=15204345, "Round Color Box 105"=15204345, "Round Color Box 106"=15204345, "Round Color Box 107"=15204345, "Round Color Box 108"=15204345, "Round Color Box 109"=15204345, "Round Color Box 110"=15204345, "Round Color Box 111"=15204345, "Round Color Box 112"=15204345, "Round Color Box 113"=15204345, "Round Color Box 114"=15204345, "Round Color Box 115"=15204345, "Round Color Box 116"=15204345, "Round Color Box 117"=15204345, "Round Color Box 118"=15204345, "Round Color Box 119"=15204345, "Round Color Box 120"=15204345, "Round Color Box 121"=15204345, "Round Color Box 122"=15204345, "Round Color Box 123"=15204345, "Round Color Box 124"=15204345, "Round Color Box 125"=15204345, "Round Color Box 126"=15204345, "Round Color Box 127"=15204345, "Round Color Box 128"=15204345, "Round Color Box 129"=15204345, "Round Color Box 130"=15204345, "Round Color Box 131"=15204345, "Round Color Box 132"=15204345, "Round Color Box 133"=15204345, "Round Color Box 134"=15204345, "Round Color Box 135"=15204345, "Round Color Box 136"=15204345, "Round Color Box 137"=15204345, "Round Color Box 138"=15204345, "Round Color Box 139"=15204345, "Round Color Box 140"=15204345, "Round Color Box 141"=15204345, "Round Color Box 142"=15204345, "Round Color Box 143"=15204345, "Round Color Box 144"=15204345, "Round Color Box 145"=15204345, "Round Color Box 146"=15204345, "Round Color Box 147"=15204345, "Round Color Box 148"=15204345, "Round Color Box 149"=15204345, "Round Color Box 150"=15204345, "Round Color Box 151"=15204345, "Round Color Box 152"=15204345, "Round Color Box 153"=15204345, "Round Color Box 154"=15204345, "Round Color Box 155"=15204345, "Round Color Box 156"=15204345, "Round Color Box 157"=15204345, "Round Color Box 158"=15204345, "Round Color Box 159"=15204345, "Round Color Box 160"=15204345, "Round Color Box 161"=15204345, "Round Color Box 162"=15204345, "Round Color Box 163"=15204345, "Round Color Box 164"=15204345, "Round Color Box 165"=15204345, "Round Color Box 166"=15204345, "Round Color Box 167"=15204345, "Round Color Box 168"=15204345, "Round Color Box 169"=15204345, "Round Color Box 170"=15204345, "Round Color Box 171"=15204345, "Round Color Box 172"=15204345, "Round Color Box 173"=15204345, "Round Color Box 174"=15204345, "Round Color Box 175"=15204345, "Round Color Box 176"=15204345} ("Cluster 2"), x=w237) -> (*(type *) &x=→"Cluster 2":T6)
        n98 = local read "stop"() -> (w236:bool)
        n99 = Wait (ms)(milliseconds to wait=u32 80) -> ()  [unwired: 1 out]
      }
      n100 = while {
        shift-right: [w212] -> _
        shift-left: w180 -> [w215]
        i -> [w214]
        stop <- w210 stop-if-true
        n101 = Equal To 0?(x=w214) -> (x = 0?=w213:bool)
        n102 = case shown="False" w213 {
          tunnel: [w217 w219] -> w212
          tunnel: w215 -> [w218 w219]
          frame False {
            n103 = Rotate 1D Array(1:w218, 2:1 ("n")) -> (0:w217:u32[])
          }
          frame True {
          }
        }
        n104 = Array To Cluster(array=w212) -> (cluster=w211:T11)
        n105 = Type Cast(type=T3 {"Round Color Box 60"=15204345, "Round Color Box 59"=15204345, "Round Color Box 58"=15204345, "Round Color Box 57"=15204345, "Round Color Box 56"=15204345, "Round Color Box 55"=15204345, "Round Color Box 54"=15204345, "Round Color Box 53"=15204345, "Round Color Box 52"=15204345, "Round Color Box 51"=15204345, "Round Color Box 50"=15204345, "Round Color Box 49"=15204345, "Round Color Box 64"=15204345, "Round Color Box 63"=15204345, "Round Color Box 62"=15204345, "Round Color Box 61"=15204345, "Round Color Box 65"=15204345, "Round Color Box 66"=15204345, "Round Color Box 67"=15204345, "Round Color Box 68"=15204345, "Round Color Box 69"=15204345, "Round Color Box 70"=15204345, "Round Color Box 71"=15204345, "Round Color Box 72"=15204345, "Round Color Box 73"=15204345, "Round Color Box 74"=15204345, "Round Color Box 75"=15204345, "Round Color Box 76"=15204345, "Round Color Box 77"=15204345, "Round Color Box 78"=15204345, "Round Color Box 79"=15204345, "Round Color Box 80"=15204345, "Round Color Box 81"=15204345, "Round Color Box 82"=15204345, "Round Color Box 83"=15204345, "Round Color Box 84"=15204345, "Round Color Box 85"=15204345, "Round Color Box 86"=15204345, "Round Color Box 87"=15204345, "Round Color Box 88"=15204345, "Round Color Box 89"=15204345, "Round Color Box 90"=15204345, "Round Color Box 91"=15204345, "Round Color Box 92"=15204345, "Round Color Box 93"=15204345, "Round Color Box 94"=15204345, "Round Color Box 95"=15204345, "Round Color Box 96"=15204345, "Round Color Box 97"=15204345, "Round Color Box 98"=15204345, "Round Color Box 99"=15204345, "Round Color Box 100"=15204345, "Round Color Box 101"=15204345, "Round Color Box 102"=15204345, "Round Color Box 103"=15204345, "Round Color Box 104"=15204345, "Round Color Box 105"=5876991, "Round Color Box 106"=47871, "Round Color Box 107"=5887743, "Round Color Box 108"=10542847, "Round Color Box 109"=13629695, "Round Color Box 110"=15204345, "Round Color Box 111"=15204345, "Round Color Box 112"=15204345, "Round Color Box 113"=15204345, "Round Color Box 114"=15204345, "Round Color Box 115"=15204345, "Round Color Box 116"=15204345, "Round Color Box 117"=15204345, "Round Color Box 118"=15204345, "Round Color Box 119"=15204345, "Round Color Box 120"=15204345, "Round Color Box 121"=15204345, "Round Color Box 122"=15204345, "Round Color Box 123"=15204345, "Round Color Box 124"=15204345, "Round Color Box 125"=15204345, "Round Color Box 126"=15204345, "Round Color Box 127"=15204345, "Round Color Box 128"=15204345, "Round Color Box 129"=15204345, "Round Color Box 130"=15204345, "Round Color Box 131"=15204345, "Round Color Box 132"=15204345, "Round Color Box 133"=15204345, "Round Color Box 134"=15204345, "Round Color Box 135"=15204345, "Round Color Box 136"=15204345, "Round Color Box 137"=15204345, "Round Color Box 138"=15204345, "Round Color Box 139"=15204345, "Round Color Box 140"=15204345, "Round Color Box 141"=15204345, "Round Color Box 142"=15204345, "Round Color Box 143"=15204345, "Round Color Box 144"=15204345, "Round Color Box 145"=15204345, "Round Color Box 146"=15204345, "Round Color Box 147"=15204345, "Round Color Box 148"=15204345, "Round Color Box 149"=15204345, "Round Color Box 150"=15204345, "Round Color Box 151"=15204345, "Round Color Box 152"=15204345, "Round Color Box 153"=15204345, "Round Color Box 154"=15204345, "Round Color Box 155"=15204345, "Round Color Box 156"=15204345, "Round Color Box 157"=15204345, "Round Color Box 158"=15204345, "Round Color Box 159"=15204345, "Round Color Box 160"=15204345, "Round Color Box 161"=15204345, "Round Color Box 162"=15204345, "Round Color Box 163"=15204345, "Round Color Box 164"=15204345, "Round Color Box 165"=15204345, "Round Color Box 166"=15204345, "Round Color Box 167"=15204345, "Round Color Box 168"=15204345, "Round Color Box 169"=15204345, "Round Color Box 170"=15204345, "Round Color Box 171"=15204345, "Round Color Box 172"=15204345, "Round Color Box 173"=15204345, "Round Color Box 174"=15204345, "Round Color Box 175"=15204345, "Round Color Box 176"=15204345} ("Cluster 3"), x=w211) -> (*(type *) &x=→"Cluster 3":T3)
        n106 = local read "stop"() -> (w210:bool)
        n107 = Wait (ms)(milliseconds to wait=u32 40) -> ()  [unwired: 1 out]
      }
      n108 = while {
        shift-right: [w199] -> _
        shift-left: w180 -> [w202]
        i -> [w201]
        stop <- w197 stop-if-true
        n109 = Equal To 0?(x=w201) -> (x = 0?=w200:bool)
        n110 = case shown="False" w200 {
          tunnel: [w204 w206] -> w199
          tunnel: w202 -> [w205 w206]
          frame False {
            n111 = Rotate 1D Array(1:w205, 2:1 ("n")) -> (0:w204:u32[])
          }
          frame True {
          }
        }
        n112 = Array To Cluster(array=w199) -> (cluster=w198:T11)
        n113 = Type Cast(type=T3 {"Round Color Box 60"=15204345, "Round Color Box 59"=15204345, "Round Color Box 58"=15204345, "Round Color Box 57"=15204345, "Round Color Box 56"=15204345, "Round Color Box 55"=15204345, "Round Color Box 54"=15204345, "Round Color Box 53"=15204345, "Round Color Box 52"=15204345, "Round Color Box 51"=15204345, "Round Color Box 50"=15204345, "Round Color Box 49"=15204345, "Round Color Box 64"=15204345, "Round Color Box 63"=15204345, "Round Color Box 62"=15204345, "Round Color Box 61"=15204345, "Round Color Box 65"=15204345, "Round Color Box 66"=15204345, "Round Color Box 67"=15204345, "Round Color Box 68"=15204345, "Round Color Box 69"=15204345, "Round Color Box 70"=15204345, "Round Color Box 71"=15204345, "Round Color Box 72"=15204345, "Round Color Box 73"=15204345, "Round Color Box 74"=15204345, "Round Color Box 75"=15204345, "Round Color Box 76"=15204345, "Round Color Box 77"=15204345, "Round Color Box 78"=15204345, "Round Color Box 79"=15204345, "Round Color Box 80"=15204345, "Round Color Box 81"=15204345, "Round Color Box 82"=15204345, "Round Color Box 83"=15204345, "Round Color Box 84"=15204345, "Round Color Box 85"=15204345, "Round Color Box 86"=15204345, "Round Color Box 87"=15204345, "Round Color Box 88"=15204345, "Round Color Box 89"=15204345, "Round Color Box 90"=15204345, "Round Color Box 91"=15204345, "Round Color Box 92"=15204345, "Round Color Box 93"=15204345, "Round Color Box 94"=15204345, "Round Color Box 95"=15204345, "Round Color Box 96"=15204345, "Round Color Box 97"=15204345, "Round Color Box 98"=15204345, "Round Color Box 99"=15204345, "Round Color Box 100"=15204345, "Round Color Box 101"=5876991, "Round Color Box 102"=47871, "Round Color Box 103"=5887743, "Round Color Box 104"=10542847, "Round Color Box 105"=13629695, "Round Color Box 106"=15204345, "Round Color Box 107"=15204345, "Round Color Box 108"=15204345, "Round Color Box 109"=15204345, "Round Color Box 110"=15204345, "Round Color Box 111"=15204345, "Round Color Box 112"=15204345, "Round Color Box 113"=15204345, "Round Color Box 114"=15204345, "Round Color Box 115"=15204345, "Round Color Box 116"=15204345, "Round Color Box 117"=15204345, "Round Color Box 118"=15204345, "Round Color Box 119"=15204345, "Round Color Box 120"=15204345, "Round Color Box 121"=15204345, "Round Color Box 122"=15204345, "Round Color Box 123"=15204345, "Round Color Box 124"=15204345, "Round Color Box 125"=15204345, "Round Color Box 126"=15204345, "Round Color Box 127"=15204345, "Round Color Box 128"=15204345, "Round Color Box 129"=15204345, "Round Color Box 130"=15204345, "Round Color Box 131"=15204345, "Round Color Box 132"=15204345, "Round Color Box 133"=15204345, "Round Color Box 134"=15204345, "Round Color Box 135"=15204345, "Round Color Box 136"=15204345, "Round Color Box 137"=15204345, "Round Color Box 138"=15204345, "Round Color Box 139"=15204345, "Round Color Box 140"=15204345, "Round Color Box 141"=15204345, "Round Color Box 142"=15204345, "Round Color Box 143"=15204345, "Round Color Box 144"=15204345, "Round Color Box 145"=15204345, "Round Color Box 146"=15204345, "Round Color Box 147"=15204345, "Round Color Box 148"=15204345, "Round Color Box 149"=15204345, "Round Color Box 150"=15204345, "Round Color Box 151"=15204345, "Round Color Box 152"=15204345, "Round Color Box 153"=15204345, "Round Color Box 154"=15204345, "Round Color Box 155"=15204345, "Round Color Box 156"=15204345, "Round Color Box 157"=15204345, "Round Color Box 158"=15204345, "Round Color Box 159"=15204345, "Round Color Box 160"=15204345, "Round Color Box 161"=15204345, "Round Color Box 162"=15204345, "Round Color Box 163"=15204345, "Round Color Box 164"=15204345, "Round Color Box 165"=15204345, "Round Color Box 166"=15204345, "Round Color Box 167"=15204345, "Round Color Box 168"=15204345, "Round Color Box 169"=15204345, "Round Color Box 170"=15204345, "Round Color Box 171"=15204345, "Round Color Box 172"=15204345, "Round Color Box 173"=15204345, "Round Color Box 174"=15204345, "Round Color Box 175"=15204345, "Round Color Box 176"=15204345} ("Cluster 9"), x=w198) -> (*(type *) &x=→"Cluster 9":T3)
        n114 = local read "stop"() -> (w197:bool)
        n115 = Wait (ms)(milliseconds to wait=u32 40) -> ()  [unwired: 1 out]
      }
      n116 = while {
        shift-right: [w186] -> _
        shift-left: w180 -> [w189]
        i -> [w188]
        stop <- w184 stop-if-true
        n117 = Equal To 0?(x=w188) -> (x = 0?=w187:bool)
        n118 = case shown="False" w187 {
          tunnel: [w191 w193] -> w186
          tunnel: w189 -> [w192 w193]
          frame False {
            n119 = Rotate 1D Array(1:w192, 2:1 ("n")) -> (0:w191:u32[])
          }
          frame True {
          }
        }
        n120 = Array To Cluster(array=w186) -> (cluster=w185:T11)
        n121 = Type Cast(type=T4 {"Round Color Box 72"=15204345, "Round Color Box 73"=15204345, "Round Color Box 74"=15204345, "Round Color Box 75"=15204345, "Round Color Box 76"=15204345, "Round Color Box 77"=15204345, "Round Color Box 78"=15204345, "Round Color Box 79"=15204345, "Round Color Box 80"=15204345, "Round Color Box 65"=15204345, "Round Color Box 66"=15204345, "Round Color Box 67"=15204345, "Round Color Box 68"=15204345, "Round Color Box 69"=15204345, "Round Color Box 70"=15204345, "Round Color Box 71"=15204345, "Round Color Box 81"=15204345, "Round Color Box 82"=15204345, "Round Color Box 83"=15204345, "Round Color Box 84"=15204345, "Round Color Box 85"=15204345, "Round Color Box 86"=15204345, "Round Color Box 87"=15204345, "Round Color Box 88"=15204345, "Round Color Box 89"=15204345, "Round Color Box 90"=15204345, "Round Color Box 91"=15204345, "Round Color Box 92"=15204345, "Round Color Box 93"=15204345, "Round Color Box 94"=15204345, "Round Color Box 95"=15204345, "Round Color Box 96"=15204345, "Round Color Box 97"=15204345, "Round Color Box 98"=15204345, "Round Color Box 99"=15204345, "Round Color Box 100"=15204345, "Round Color Box 101"=15204345, "Round Color Box 102"=15204345, "Round Color Box 103"=15204345, "Round Color Box 104"=15204345, "Round Color Box 105"=15204345, "Round Color Box 106"=15204345, "Round Color Box 107"=15204345, "Round Color Box 108"=15204345, "Round Color Box 109"=15204345, "Round Color Box 110"=15204345, "Round Color Box 111"=15204345, "Round Color Box 112"=15204345, "Round Color Box 113"=15204345, "Round Color Box 114"=15204345, "Round Color Box 115"=15204345, "Round Color Box 116"=15204345, "Round Color Box 117"=5876991, "Round Color Box 118"=47871, "Round Color Box 119"=5887743, "Round Color Box 120"=10542847, "Round Color Box 121"=13629695, "Round Color Box 122"=15204345, "Round Color Box 123"=15204345, "Round Color Box 124"=15204345, "Round Color Box 125"=15204345, "Round Color Box 126"=15204345, "Round Color Box 127"=15204345, "Round Color Box 128"=15204345, "Round Color Box 129"=15204345, "Round Color Box 130"=15204345, "Round Color Box 131"=15204345, "Round Color Box 132"=15204345, "Round Color Box 133"=15204345, "Round Color Box 134"=15204345, "Round Color Box 135"=15204345, "Round Color Box 136"=15204345, "Round Color Box 137"=15204345, "Round Color Box 138"=15204345, "Round Color Box 139"=15204345, "Round Color Box 140"=15204345, "Round Color Box 141"=15204345, "Round Color Box 142"=15204345, "Round Color Box 143"=15204345, "Round Color Box 144"=15204345, "Round Color Box 145"=15204345, "Round Color Box 146"=15204345, "Round Color Box 147"=15204345, "Round Color Box 148"=15204345, "Round Color Box 149"=15204345, "Round Color Box 150"=15204345, "Round Color Box 151"=15204345, "Round Color Box 152"=15204345, "Round Color Box 153"=15204345, "Round Color Box 154"=15204345, "Round Color Box 155"=15204345, "Round Color Box 156"=15204345, "Round Color Box 157"=15204345, "Round Color Box 158"=15204345, "Round Color Box 159"=15204345, "Round Color Box 160"=15204345, "Round Color Box 161"=15204345, "Round Color Box 162"=15204345, "Round Color Box 163"=15204345, "Round Color Box 164"=15204345, "Round Color Box 165"=15204345, "Round Color Box 166"=15204345, "Round Color Box 167"=15204345, "Round Color Box 168"=15204345, "Round Color Box 169"=15204345, "Round Color Box 170"=15204345, "Round Color Box 171"=15204345, "Round Color Box 172"=15204345, "Round Color Box 173"=15204345, "Round Color Box 174"=15204345, "Round Color Box 175"=15204345, "Round Color Box 176"=15204345, "Round Color Box 177"=15204345, "Round Color Box 178"=15204345, "Round Color Box 179"=15204345, "Round Color Box 180"=15204345, "Round Color Box 181"=15204345, "Round Color Box 182"=15204345, "Round Color Box 183"=15204345, "Round Color Box 184"=15204345, "Round Color Box 185"=15204345, "Round Color Box 186"=15204345, "Round Color Box 187"=15204345, "Round Color Box 188"=15204345, "Round Color Box 189"=15204345, "Round Color Box 190"=15204345, "Round Color Box 191"=15204345, "Round Color Box 192"=15204345} ("Cluster 10"), x=w185) -> (*(type *) &x=→"Cluster 10":T4)
        n122 = local read "stop"() -> (w184:bool)
        n123 = Wait (ms)(milliseconds to wait=u32 40) -> ()  [unwired: 1 out]
      }
    }
    frame Enabled {
    }
  }
  n124 = disable-structure shown="Disabled" {
    frame Disabled {
      n125 = call <vilib>:"RGB to Color.vi"() -> ()  [unwired: 3 in, 1 out]
    }
    frame Enabled {
    }
  }
